vi "Auth Method.vi"(11 "WampScramAuthenticator in":refnum<class "WampScramAuthenticator.lvclass">) -> (2 "Authmethod":string, 3 "WampScramAuthenticator out":refnum<class "WampScramAuthenticator.lvclass">)   [LabVIEW 2020, in "wamplv.lvlib" / "WampScramAuthenticator.lvclass"]
uses:
  WampScramAuthenticator.lvclass
  WampScramAuthenticator.lvclass/WampScramAuthenticator.ctl
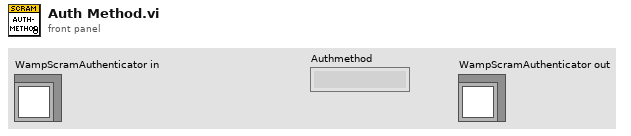
[diagram p1: front panel]
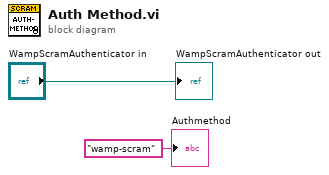
[diagram p0: block diagram]
diagram:
  "WampScramAuthenticator out" <- "WampScramAuthenticator in"
  "Authmethod" <- "wamp-scram" ("Authmethod")
